vi "Set_Parameter_Row_tl.vi"(4 "Parameter Row":string[][](table)) -> (0 "PARAMETERS\nWRITTEN OK?":bool)   [LabVIEW 2010]
doc: "This VI sets the PRO-J positioner's parameter table using a single row of parameters held in the Macintosh"
panel:
  out "to value":string
  out "Currently setting":string
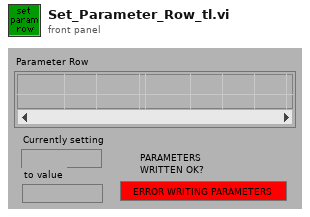
[diagram p1: front panel]
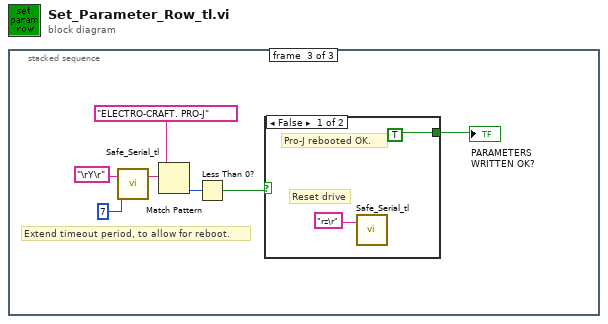
[diagram p0: block diagram]
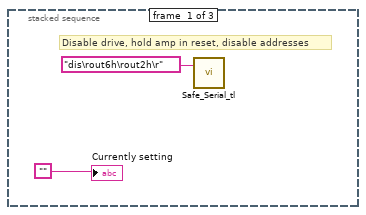
[diagram p2: hidden frame]
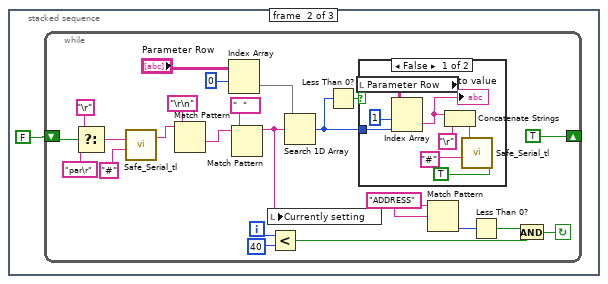
[diagram p3: hidden frame]
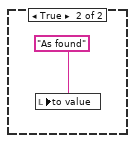
[diagram p4: hidden frame]
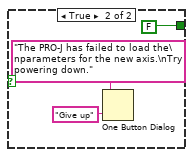
[diagram p5: hidden frame]
diagram:
  n1 = stacked-sequence {
    frame #0 {
      # "Disable drive, hold amp in reset, disable addresses"
      n2 = call "Safe_Serial_tl.vi"("Tx String"="dis\rout6h\rout2h\r") -> ()  [unwired: 5 in, 2 out]
      "Currently setting" <- ""
    }
    frame #1 {
      n3 = while {
        shift-left: FALSE -> [w25]
        shift-right: [TRUE] -> _
        i -> [w9]
        stop <- w11 continue-if-true
        n4 = Select(t="\r", s=w25, f="par\r") -> (s? t:f=w6:string)
        n5 = call "Safe_Serial_tl.vi"("Tx String"=w6, "Terminator (glob)"="#") -> ("Rx String"=w4:string)  [unwired: 4 in, 1 out]
        n6 = Match Pattern(string=w4, regular expression="\r\n") -> (after substring=w21:string)  [unwired: 1 in, 3 out]
        n7 = Index Array(array="Parameter Row", index (row)=0) -> (element=w17:string[])  [unwired: 1 in]
        n8 = Match Pattern(string=w21, regular expression="  ") -> (before substring=w14:string)  [unwired: 1 in, 3 out]
        n9 = local write "Currently setting"(w14) -> ()
        n10 = Less?(x=w9, y=40) -> (x < y?=w7:bool)
        n11 = Search 1D Array(1D array=w17, element=w14) -> (index of element=w19:i32)  [unwired: 1 in]
        n12 = Less Than 0?(x=w19) -> (x < 0?=w20:bool)
        n13 = case shown="False" w20 {
          tunnel: w19 -> [w31 _]
          frame False {
            n14 = local read "Parameter Row"() -> (w34:string[][])
            n15 = Index Array(array=w34, index (row)=1, index (col)=w31) -> (element=w29:string)
            "to value" <- w29
            n16 = Concatenate Strings(w29, "\r") -> (w33:string)
            n17 = call "Safe_Serial_tl.vi"("Tx String"=w33, "Terminator (glob)"="#", "Echo Checking (F)"=TRUE) -> ()  [unwired: 3 in, 2 out]
          }
          frame True {
            n18 = local write "to value"("As found") -> ()
          }
        }
        n19 = Match Pattern(string=w14, regular expression="ADDRESS") -> (offset past match=w13:i32)  [unwired: 1 in, 3 out]
        n20 = Less Than 0?(x=w13) -> (x < 0?=w10:bool)
        n21 = And(x=w10, y=w7) -> (x .and. y?=w11:bool)
      }
    }
    frame #2 {
      # "Extend timeout period, to allow for reboot."
      n22 = call "Safe_Serial_tl.vi"("Tx String"="\rY\r", "Timeout (glob)"=7) -> ("Rx String"=w39:string)  [unwired: 4 in, 1 out]
      n23 = Match Pattern(string=w39, regular expression="ELECTRO-CRAFT. PRO-J") -> (offset past match=w38:i32)  [unwired: 1 in, 3 out]
      n24 = Less Than 0?(x=w38) -> (x < 0?=w40:bool)
      n25 = case shown="False" w40 {
        tunnel: [TRUE FALSE] -> w37
        frame False {
          # "Reset drive"
          # "Pro-J rebooted OK."
          n26 = call "Safe_Serial_tl.vi"("Tx String"="rz\r") -> ()  [unwired: 5 in, 2 out]
        }
        frame True {
          n27 = One Button Dialog(message="The PRO-J has failed to load the\nparameters for the new axis.\nTry powering down.", button name ("OK")="Give up") -> ()  [unwired: 1 out]
        }
      }
      "PARAMETERS\nWRITTEN OK?" <- w37
    }
  }
